vi "File or directory exists.vi"(8 "error in (no error)":errorcluster, 10 "Path":string, 11 "SCP File Transfer in":refnum<class "SCP File Transfer.lvclass">) -> (0 "error out":errorcluster, 1 "Exists?":bool, 2 "Path out (dup)":string, 3 "SCP File Transfer out":refnum<class "SCP File Transfer.lvclass">, 4 "Type":T1)   [LabVIEW 2014, in "PL Framework Configuration Tool.lvlib" / "SCP File Transfer.lvclass"]
doc: "Checks to see if the file or directory at \"Path\" exists or not.\n\nThe recommended file path format for \"Path\" is \"/directory1/directory2\" or \"/directory/file.extension\". However, the VI will accept other formats and transform the path appropriately in most cases. Use the \"Strip path.vi\" and \"Build path.vi\" VIs to help with handling remote path strings."
uses:
  <vilib>/NI/DCAF/Tag Editor Core/Configuration Editor/Classes/Deployment Helpers/SCP File Transfer/SCP File Transfer.lvclass
  <vilib>/NI/RT Management/classes/File Transfer Behavior/Type.ctl
  <vilib>/NI/DCAF/Tag Editor Core/Configuration Editor/Classes/Deployment Helpers/SCP File Transfer/SCP File Transfer.lvclass/SCP File Transfer.ctl
  <vilib>/NI/RT Management/classes/File Transfer Behavior/File Transfer Behavior.lvclass
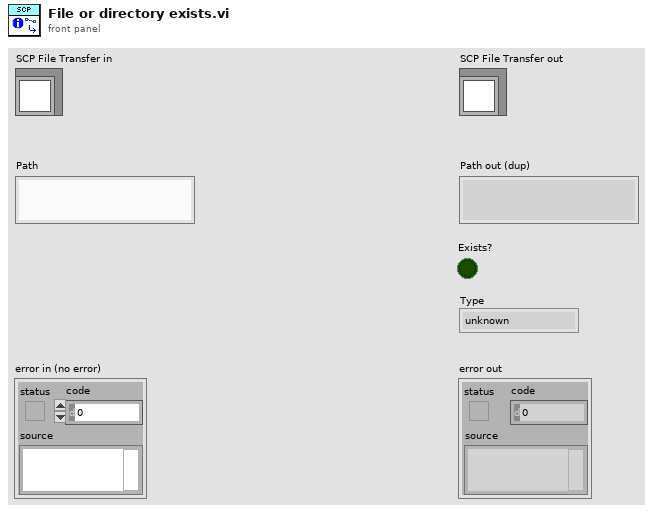
[diagram p1: front panel]
types:
  T1 = typedef "RT Management.lvlib/File Transfer Behavior.lvclass/Type.ctl" = enum16{"unknown", "file", "directory"}
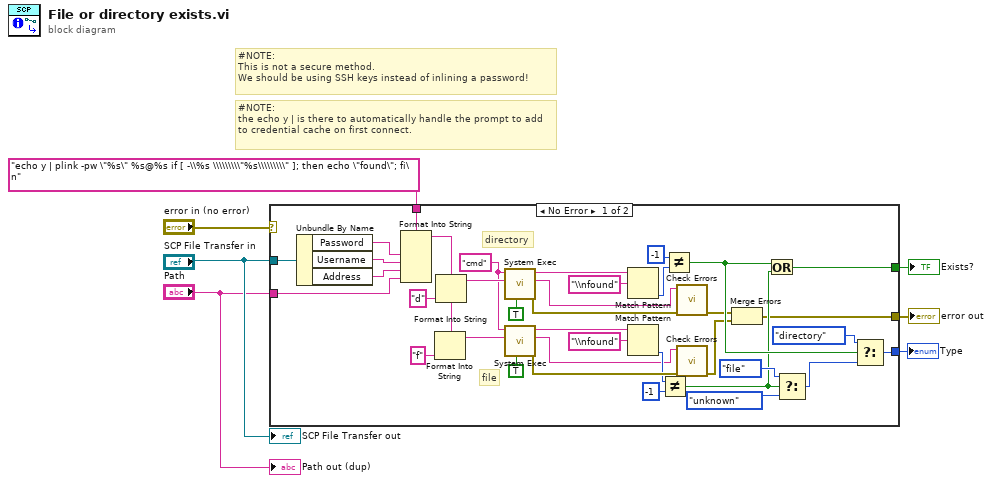
[diagram p0: block diagram]
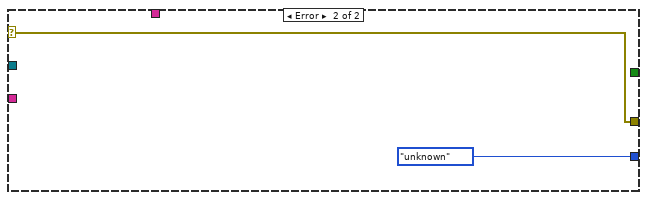
[diagram p2: hidden frame]
diagram:
  # "#NOTE:\nthe echo y | is there to automatically handle the prompt to add to credential cache on first connect."
  # "#NOTE:\nThis is not a secure method.\nWe should be using SSH keys instead of inlining a password!"
  n1 = case shown="No Error" "error in (no error)" {
    selector: "error in (no error)" -> [_ w45]
    tunnel: "echo y | plink -pw \"%s\" %s@%s if [ -\\%s \\\\\\\\\"%s\\\\\\\\\" ]; then echo \"found\"; fi\n" ("format string") -> [w40 _]
    tunnel: "Path" -> [w36 _]
    tunnel: "SCP File Transfer in" -> [w41 _]
    tunnel: [w10 w45] -> w5
    tunnel: [w30 _] -> w2
    tunnel: [w29 Type."unknown" ("Type 2")] -> w1
    frame No Error {
      w19 = "cmd" ("command line")
      # "file"
      # "directory"
      n2 = Unbundle By Name(w41) -> ("Password"=w39:string, "Username"=w38:string, "Address"=w37:string)
      n3 = Format Into String(format string=w40, w39, w38, w37, w36) -> (resulting string=w28:string)  [unwired: 2 in, 1 out]
      n4 = Format Into String(format string=w28, "f" ("input 1")) -> (resulting string=w20:string)  [unwired: 2 in, 1 out]
      n5 = Format Into String(format string=w28, "d" ("input 1")) -> (resulting string=w25:string)  [unwired: 2 in, 1 out]
      n6 = call <vilib>:"System Exec.vi"("run minimized? (F)"=TRUE, "standard input"=w25, "command line"=w19) -> ("error out"=w44:errorcluster, "standard error"=w13:string, "standard output"=w42:string)  [unwired: 5 in, 1 out]
      n7 = call <vilib>:"System Exec.vi"("run minimized? (F)"=TRUE, "standard input"=w20, "command line"=w19) -> ("error out"=w22:errorcluster, "standard error"=w12:string, "standard output"=w24:string)  [unwired: 5 in, 1 out]
      n8 = Match Pattern(string=w42, regular expression="\\nfound") -> (offset past match=w16:i32)  [unwired: 1 in, 3 out]
      n9 = Match Pattern(string=w24, regular expression="\\nfound") -> (offset past match=w17:i32)  [unwired: 1 in, 3 out]
      n10 = Not Equal?(x=w17, y=-1) -> (x != y?=w14:bool)
      n11 = Not Equal?(x=-1 ("y"), y=w16) -> (x != y?=w31:bool)
      n12 = call <vilib>:"Check Errors.vi"("error in (no error)"=w44, "standard error"=w13) -> ("error out"=w11:errorcluster)  [unwired: 9 in]
      n13 = call <vilib>:"Check Errors.vi"("error in (no error)"=w22, "standard error"=w12) -> ("error out"=w9:errorcluster)  [unwired: 9 in]
      n14 = Merge Errors(w11, w9) -> (w10:errorcluster)
      n15 = Or(x=w31, y=w14) -> (x .or. y?=w30:bool)
      n16 = Select(t=Type."file" ("Type 2"), s=w14, f=Type."unknown" ("Type 2")) -> (s? t:f=w33:T1)
      n17 = Select(t=Type."directory" ("Type 2"), s=w31, f=w33) -> (s? t:f=w29:T1)
    }
    frame Error {
    }
  }
  "error out" <- w5
  "Exists?" <- w2
  "Type" <- w1
  "SCP File Transfer out" <- "SCP File Transfer in"
  "Path out (dup)" <- "Path"
